vi "ADC Initialize Virtual Channels.vi"(8 "error in":errorcluster, 10 "Reset? (False)":bool, 11 "adc session in":T1={"niScope"={"channel cfg"=[], "sessions"=[], "multi cards"=FALSE, "channels"=0, "type"=enum."n/a", "memory [B/chn]"=0, "ext. clock [Hz]"=0.0, "samples count"=0, "use streaming"=FALSE, "proc setup"={"packet size [smpl]"=0, "current timeout [s]"=0.0, "blk2blk timeout [s]"=0.0, "event time"=timestamp(0 s since 1904-01-01), "temp sampl T [s]"=0.0, "data queue"=refnum, "stop notifier"=refnum, "proc ref"=refnum}, "sample width [B]"=0, "ranges [V]"=[], "trigger setup"={"coupling"=1, "level [V]"=0.0, "slope"=0, "mode"=enum."Immediate", "pre-trigger [%]"=0.0}, "fs [Hz]"=0.0, "bitres [bit]"=0, "clock source"=enum."VAL_NO_SOURCE"}, "3458A"={"channels"=[], "sync unit"={"VISA"="", "type"=enum."Picotest U6200A"}, "awg unit"={"type"=enum."Agilent 331xxA to 332xxA", "VISA"="", "enable 10MHz ref"=FALSE, "cmi ckd2"={"VISA"="", "clock source"=enum."Auto", "manual ref clk"=FALSE, "ref clock [Hz]"=0.0, "div mode"=enum."Set divisor directly"}, "cmi sync v3"={"VISA"="", "baud rate [bd/s]"=115200, "source"=enum."Auto", "hv range"=enum."1kV", "fsrc is fixed"=FALSE, "fsrc [Hz]"=10000000.0, "freq integ [s]"=1.0, "freq filter"=5, "trig level"=enum."TTL 5V", "chn1 mode"=enum."Source divider", "chn1 level"=enum."Positive 5V", "chn2 mode"=enum."Source divider", "chn2 level"=enum."Positive 5V", "chn2 div"=1, "chn3 mode"=enum."Chn 1 Active", "chn3 level"=enum."Positive 5V", "chn1 div entry"=enum."Calculate nearest divisor from measured fx", "chn1 dev limit [%]"=1.0, "chn1 check dev"=FALSE}, "trigger"={"source"=enum."Immediate", "slope"=enum."POS", "coupling"=enum."DC", "level [V]"=0.0, "hysteresis [V]"=0.0, "pre-trigger [%]"=0.0}, "HMF2500 cfg"={"Baud Rate"=9600, "Parity"=0, "Data Bits"=8, "Flow Control"=4}}, "sync mode"=enum."MASTER-SLAVE, MASTER clocked by TIMER", "streaming mode"=FALSE, "idn mode"=enum."Auto", "sampling mode"=enum."DCV", "sample memory [B]"=0, "proc setup"={"channel id"=0, "packet size [smpl]"=0, "current timeout [s]"=0.0, "blk2blk timeout [s]"=0.0, "event time"=timestamp(0 s since 1904-01-01), "stop notifier"=refnum, "data queues"=[], "proc refs"=[], "bus semaphore"=refnum}, "sample size [B]"=0, "sample count"=0, "aux data"={"channel id"=0, "valid?"=[], "gain [V]"=[], "timestamp [s]"=[], "Ts [s]"=0.0, "abs timestamp"=timestamp(0 s since 1904-01-01), "t [deg C]"=[], "multiplex timestamp [s]"=-1.0, "only multiplex?"=FALSE, "multiplex smpl offset"=0, "overflow?"=FALSE}, "ranges [V]"=[], "aperture [s]"=0.0, "LEVEL trigger"={"edge"=enum."POS", "level [V]"=0.0, "coupling"=enum."DC"}, "trigger mode"=enum."AUTO", "measure temp.?"=FALSE, "disp mesages"=[], "shared bus?"=FALSE, "disable display?"=FALSE, "aper mode"=enum."Manual", "aper rules"=[], "multiplex"={"cycles"=0, "delay [s]"=0.0, "enabled"=FALSE, "overhead [s]"=1.0, "tot smpls"=0, "sub-rec"=0, "overhead [%]"=0.0, "emulated"=FALSE}, "F8588 lpf"=enum."Off", "F8588 pll"=enum."Off", "F8588 couple"=enum."DC, auto", "fs"={"freq mode"=enum."fs or Ts", "fs [Hz]"=0.0, "fref [Hz]"=0.0, "mul"=0.0, "div"=0.0}, "fs mode"=enum."fs or Ts"}, "dsdll"={"dsdll"={"dsdll path"=path "", "dsdll handle"=[], "output devices"=[], "capture devices"=[]}, "channels"=0, "device id"=0, "channel idns"=[], "proc setup"={"packet size [smpl]"=0, "current timeout [s]"=0.0, "blk2blk timeout [s]"=0.0, "event time"=timestamp(0 s since 1904-01-01), "data queue"=refnum, "stop notifier"=refnum, "proc ref"=refnum}, "samples count"=0, "fs [Hz]"=0.0}, "type"=enum."niScope", "channel idn str"=[], "aux instr idn str"=[], "modified?"=FALSE, "simadc"={"channels"=[], "range [V]"=0.0, "Ts step [s]"=0.0, "time [s]"=0.0, "fs [Hz]"=0.0, "count"=0, "smpl offset"=0, "set count"=0, "bit res"=0}, "force rst?"=FALSE, "exit mode"=enum."Immediate reset", "exit dly"=0.0, "exit tmr"=timestamp(0 s since 1904-01-01), "busy?"=FALSE, "accessed?"=FALSE, "multiplex"={"Type"=enum."Dummy", "gen com ssn"={"visa"="", "primary"=enum."None", "secondary"=enum."None", "channels"=[]}, "delay before [s]"=0.0, "delay post [s]"=0.0, "sequence"=[], "enabled"=FALSE, "ref timestamp [s]"=0.0, "idn string"="", "dev niScope"="", "niScope idx"=0, "QPMX ssn"={"visa"="", "switch mode"=enum."Switched by TWM", "sequence"=[], "timing delays"=[], "polarity"=enum."Positive", "ss delay (s)"=2.0, "internal timer (s)"=1.0, "Last loaded sequence file"=path "", "startup delay (s)"=2.0}, "VISA mux ssn"={"VISA"="", "paths"=[], "idn command"="", "serial cfg"={"Baud rate"=9600, "Data bits"=8, "Parity"=0, "Stop bits"=10, "Flow control"=0, "End Mode Read"=enum."None", "End Mode Write"=enum."None", "Term character"=0, "Term enable"=FALSE}}}, "keysight dso"={"VISA"="", "channels"=[], "bw limit [Hz]"=0.0, "resolution"=enum."Basic", "trig noise reject"=enum."Normal", "N"=0, "trigger config"={"trigger source"=enum."Immediate", "trigger slope"=enum."Negative", "level [V]"=0.0, "hysteresis [V]"=0.001, "pre-trig [%]"=50}, "fs [Hz]"=0.0, "timeout stop"=timestamp(0 s since 1904-01-01), "waiting for opc"=FALSE, "fetch offset [smpl]"=0, "abs timestamp"=timestamp(0 s since 1904-01-01), "ranges [V]"=[], "decimation"=1.0, "ext ref"=FALSE, "emulate aperture"=FALSE, "model"=enum."DSO91304"}, "cdaq"={"mclk [Hz]"=12800000.0, "ADC task"="", "mclk reference"="", "fs [Hz]"=50000.0, "queue adc cmd"=refnum, "queue adc data"=refnum, "adc proc ref"=refnum, "channels"=[], "last channels"=[], "timeout"=timestamp(0 s since 1904-01-01), "N"=1000, "mclk mode"=enum."Free running", "ext mclk source"=""}, "ignore overload"=FALSE, "ADS127L21"={"VISA"="", "chn list"=[], "record size"=0, "phys. channels"=0, "adc fifo size"=0, "channels"=[], "ext refclk?"=FALSE, "fs [Hz]"=0.0, "ext refclk [Hz]"=0.0, "meas refclk [Hz]"=0.0, "EXTOUT mode"=enum."ADCCLK", "EXTOUT polarity"=enum."NORM", "EXTOUT divisor"=0}} {"ADS127L21"."channels"."Channel" min=1 max=8 step=1; "cdaq"."last channels"."Channel id" min=0 step=1; "cdaq"."channels"."Channel id" min=0 step=1; "keysight dso"."decimation" min=1.0; "keysight dso"."bw limit [Hz]" format="%#_6p"; "keysight dso"."channels"."Offset [V]" format="%#_6p"; "keysight dso"."channels"."Range [Vpk]" min=0.0 format="%#_6p"; "keysight dso"."channels"."Channel" min=1; "multiplex"."VISA mux ssn"."serial cfg"."Flow control" items=["None", "XON/XOFF", "CTS/RTS", "XON/XOFF + CTS/RTS", "DTR/DSR", "XON/XOFF + DTR/DSR"]; "multiplex"."VISA mux ssn"."serial cfg"."Stop bits" items=["1 bit"=10, "1.5 bits"=15, "2 bits"=20]; "multiplex"."VISA mux ssn"."serial cfg"."Parity" items=["None", "Odd", "Even", "Mark", "Space"]; "multiplex"."VISA mux ssn"."serial cfg"."Data bits" items=["5 bits"=5, "6 bits"=6, "7 bits"=7, "8 bits"=8]; "multiplex"."VISA mux ssn"."serial cfg"."Baud rate" items=["150 Bd"=150, "300 Bd"=300, "600 Bd"=600, "1200 Bd"=1200, "2400 Bd"=2400, "4800 Bd"=4800, "9600 Bd"=9600, "19.2 kBd"=19200, "38.4 kBd"=38400, "57.6 kBd"=57600, "115.2 kBd"=115200]; "multiplex"."QPMX ssn"."startup delay (s)" min=0.0 step=1.0; "multiplex"."QPMX ssn"."internal timer (s)" min=0.0 step=1.0; "multiplex"."QPMX ssn"."ss delay (s)" min=0.0 step=1.0; "multiplex"."QPMX ssn"."timing delays" min=1 max=255 step=1; "3458A"."awg unit"."HMF2500 cfg"."Flow Control" items=["None", "XON/XOFF", "RTS/CTS", "XON/XOFF & RTS/CTS", "DTR/DSR", "XON/XOFF & DTR/DSR"]; "3458A"."awg unit"."HMF2500 cfg"."Data Bits" items=["7"=7, "8"=8]; "3458A"."awg unit"."HMF2500 cfg"."Parity" items=["None", "Odd", "Even", "Mark", "Space"]; "3458A"."awg unit"."HMF2500 cfg"."Baud Rate" items=["300"=300, "600"=600, "1200"=1200, "2400"=2400, "4800"=4800, "9600"=9600, "19200"=19200]; "3458A"."awg unit"."cmi sync v3"."chn2 div" min=1 max=100000000 step=1; "3458A"."awg unit"."cmi sync v3"."fsrc [Hz]" format="%_8p"; "3458A"."channels"."Range [Vpk]" min=0.0; "niScope"."trigger setup"."pre-trigger [%]" format="%.2f"; "niScope"."trigger setup"."level [V]" format="%.2f"; "niScope"."trigger setup"."coupling" items=["AC"=0, "DC"=1, "HF Reject"=3, "LF Reject"=4, "AC Plus HF Reject"=1001]; "niScope"."channel cfg"."Range [Vpk]" min=0.0; "niScope"."channel cfg"."Channel" min=0}) -> (0 "error out":errorcluster, 1 "aux instr. idn strings":string[](array[string]), 2 "channel idn strings":string[](array[string]), 3 "adc session out":T1={"niScope"={"channel cfg"=[], "sessions"=[], "multi cards"=FALSE, "channels"=0, "type"=enum."n/a", "memory [B/chn]"=0, "ext. clock [Hz]"=0.0, "samples count"=0, "use streaming"=FALSE, "proc setup"={"packet size [smpl]"=0, "current timeout [s]"=0.0, "blk2blk timeout [s]"=0.0, "event time"=timestamp(0 s since 1904-01-01), "temp sampl T [s]"=0.0, "data queue"=refnum, "stop notifier"=refnum, "proc ref"=refnum}, "sample width [B]"=0, "ranges [V]"=[], "trigger setup"={"coupling"=1, "level [V]"=0.0, "slope"=0, "mode"=enum."Immediate", "pre-trigger [%]"=0.0}, "fs [Hz]"=0.0, "bitres [bit]"=0, "clock source"=enum."VAL_NO_SOURCE"}, "3458A"={"channels"=[], "sync unit"={"VISA"="", "type"=enum."Picotest U6200A"}, "awg unit"={"type"=enum."Agilent 331xxA to 332xxA", "VISA"="", "enable 10MHz ref"=FALSE, "cmi ckd2"={"VISA"="", "clock source"=enum."Auto", "manual ref clk"=FALSE, "ref clock [Hz]"=0.0, "div mode"=enum."Set divisor directly"}, "cmi sync v3"={"VISA"="", "baud rate [bd/s]"=115200, "source"=enum."Auto", "hv range"=enum."1kV", "fsrc is fixed"=FALSE, "fsrc [Hz]"=10000000.0, "freq integ [s]"=1.0, "freq filter"=5, "trig level"=enum."TTL 5V", "chn1 mode"=enum."Source divider", "chn1 level"=enum."Positive 5V", "chn2 mode"=enum."Source divider", "chn2 level"=enum."Positive 5V", "chn2 div"=1, "chn3 mode"=enum."Chn 1 Active", "chn3 level"=enum."Positive 5V", "chn1 div entry"=enum."Calculate nearest divisor from measured fx", "chn1 dev limit [%]"=1.0, "chn1 check dev"=FALSE}, "trigger"={"source"=enum."Immediate", "slope"=enum."POS", "coupling"=enum."DC", "level [V]"=0.0, "hysteresis [V]"=0.0, "pre-trigger [%]"=0.0}, "HMF2500 cfg"={"Baud Rate"=9600, "Parity"=0, "Data Bits"=8, "Flow Control"=4}}, "sync mode"=enum."MASTER-SLAVE, MASTER clocked by TIMER", "streaming mode"=FALSE, "idn mode"=enum."Auto", "sampling mode"=enum."DCV", "sample memory [B]"=0, "proc setup"={"channel id"=0, "packet size [smpl]"=0, "current timeout [s]"=0.0, "blk2blk timeout [s]"=0.0, "event time"=timestamp(0 s since 1904-01-01), "stop notifier"=refnum, "data queues"=[], "proc refs"=[], "bus semaphore"=refnum}, "sample size [B]"=0, "sample count"=0, "aux data"={"channel id"=0, "valid?"=[], "gain [V]"=[], "timestamp [s]"=[], "Ts [s]"=0.0, "abs timestamp"=timestamp(0 s since 1904-01-01), "t [deg C]"=[], "multiplex timestamp [s]"=-1.0, "only multiplex?"=FALSE, "multiplex smpl offset"=0, "overflow?"=FALSE}, "ranges [V]"=[], "aperture [s]"=0.0, "LEVEL trigger"={"edge"=enum."POS", "level [V]"=0.0, "coupling"=enum."DC"}, "trigger mode"=enum."AUTO", "measure temp.?"=FALSE, "disp mesages"=[], "shared bus?"=FALSE, "disable display?"=FALSE, "aper mode"=enum."Manual", "aper rules"=[], "multiplex"={"cycles"=0, "delay [s]"=0.0, "enabled"=FALSE, "overhead [s]"=1.0, "tot smpls"=0, "sub-rec"=0, "overhead [%]"=0.0, "emulated"=FALSE}, "F8588 lpf"=enum."Off", "F8588 pll"=enum."Off", "F8588 couple"=enum."DC, auto", "fs"={"freq mode"=enum."fs or Ts", "fs [Hz]"=0.0, "fref [Hz]"=0.0, "mul"=0.0, "div"=0.0}, "fs mode"=enum."fs or Ts"}, "dsdll"={"dsdll"={"dsdll path"=path "", "dsdll handle"=[], "output devices"=[], "capture devices"=[]}, "channels"=0, "device id"=0, "channel idns"=[], "proc setup"={"packet size [smpl]"=0, "current timeout [s]"=0.0, "blk2blk timeout [s]"=0.0, "event time"=timestamp(0 s since 1904-01-01), "data queue"=refnum, "stop notifier"=refnum, "proc ref"=refnum}, "samples count"=0, "fs [Hz]"=0.0}, "type"=enum."niScope", "channel idn str"=[], "aux instr idn str"=[], "modified?"=FALSE, "simadc"={"channels"=[], "range [V]"=0.0, "Ts step [s]"=0.0, "time [s]"=0.0, "fs [Hz]"=0.0, "count"=0, "smpl offset"=0, "set count"=0, "bit res"=0}, "force rst?"=FALSE, "exit mode"=enum."Immediate reset", "exit dly"=0.0, "exit tmr"=timestamp(0 s since 1904-01-01), "busy?"=FALSE, "accessed?"=FALSE, "multiplex"={"Type"=enum."Dummy", "gen com ssn"={"visa"="", "primary"=enum."None", "secondary"=enum."None", "channels"=[]}, "delay before [s]"=0.0, "delay post [s]"=0.0, "sequence"=[], "enabled"=FALSE, "ref timestamp [s]"=0.0, "idn string"="", "dev niScope"="", "niScope idx"=0, "QPMX ssn"={"visa"="", "switch mode"=enum."Switched by TWM", "sequence"=[], "timing delays"=[], "polarity"=enum."Positive", "ss delay (s)"=2.0, "internal timer (s)"=1.0, "Last loaded sequence file"=path "", "startup delay (s)"=2.0}, "VISA mux ssn"={"VISA"="", "paths"=[], "idn command"="", "serial cfg"={"Baud rate"=9600, "Data bits"=8, "Parity"=0, "Stop bits"=10, "Flow control"=0, "End Mode Read"=enum."None", "End Mode Write"=enum."None", "Term character"=0, "Term enable"=FALSE}}}, "keysight dso"={"VISA"="", "channels"=[], "bw limit [Hz]"=0.0, "resolution"=enum."Basic", "trig noise reject"=enum."Normal", "N"=0, "trigger config"={"trigger source"=enum."Immediate", "trigger slope"=enum."Negative", "level [V]"=0.0, "hysteresis [V]"=0.001, "pre-trig [%]"=50}, "fs [Hz]"=0.0, "timeout stop"=timestamp(0 s since 1904-01-01), "waiting for opc"=FALSE, "fetch offset [smpl]"=0, "abs timestamp"=timestamp(0 s since 1904-01-01), "ranges [V]"=[], "decimation"=1.0, "ext ref"=FALSE, "emulate aperture"=FALSE, "model"=enum."DSO91304"}, "cdaq"={"mclk [Hz]"=12800000.0, "ADC task"="", "mclk reference"="", "fs [Hz]"=50000.0, "queue adc cmd"=refnum, "queue adc data"=refnum, "adc proc ref"=refnum, "channels"=[], "last channels"=[], "timeout"=timestamp(0 s since 1904-01-01), "N"=1000, "mclk mode"=enum."Free running", "ext mclk source"=""}, "ignore overload"=FALSE, "ADS127L21"={"VISA"="", "chn list"=[], "record size"=0, "phys. channels"=0, "adc fifo size"=0, "channels"=[], "ext refclk?"=FALSE, "fs [Hz]"=0.0, "ext refclk [Hz]"=0.0, "meas refclk [Hz]"=0.0, "EXTOUT mode"=enum."ADCCLK", "EXTOUT polarity"=enum."NORM", "EXTOUT divisor"=0}} {"ADS127L21"."channels"."Channel" min=1 max=8 step=1; "cdaq"."last channels"."Channel id" min=0 step=1; "cdaq"."channels"."Channel id" min=0 step=1; "keysight dso"."decimation" min=1.0; "keysight dso"."bw limit [Hz]" format="%#_6p"; "keysight dso"."channels"."Offset [V]" format="%#_6p"; "keysight dso"."channels"."Range [Vpk]" min=0.0 format="%#_6p"; "keysight dso"."channels"."Channel" min=1; "multiplex"."VISA mux ssn"."serial cfg"."Flow control" items=["None", "XON/XOFF", "CTS/RTS", "XON/XOFF + CTS/RTS", "DTR/DSR", "XON/XOFF + DTR/DSR"]; "multiplex"."VISA mux ssn"."serial cfg"."Stop bits" items=["1 bit"=10, "1.5 bits"=15, "2 bits"=20]; "multiplex"."VISA mux ssn"."serial cfg"."Parity" items=["None", "Odd", "Even", "Mark", "Space"]; "multiplex"."VISA mux ssn"."serial cfg"."Data bits" items=["5 bits"=5, "6 bits"=6, "7 bits"=7, "8 bits"=8]; "multiplex"."VISA mux ssn"."serial cfg"."Baud rate" items=["150 Bd"=150, "300 Bd"=300, "600 Bd"=600, "1200 Bd"=1200, "2400 Bd"=2400, "4800 Bd"=4800, "9600 Bd"=9600, "19.2 kBd"=19200, "38.4 kBd"=38400, "57.6 kBd"=57600, "115.2 kBd"=115200]; "multiplex"."QPMX ssn"."startup delay (s)" min=0.0 step=1.0; "multiplex"."QPMX ssn"."internal timer (s)" min=0.0 step=1.0; "multiplex"."QPMX ssn"."ss delay (s)" min=0.0 step=1.0; "multiplex"."QPMX ssn"."timing delays" min=1 max=255 step=1; "3458A"."awg unit"."HMF2500 cfg"."Flow Control" items=["None", "XON/XOFF", "RTS/CTS", "XON/XOFF & RTS/CTS", "DTR/DSR", "XON/XOFF & DTR/DSR"]; "3458A"."awg unit"."HMF2500 cfg"."Data Bits" items=["7"=7, "8"=8]; "3458A"."awg unit"."HMF2500 cfg"."Parity" items=["None", "Odd", "Even", "Mark", "Space"]; "3458A"."awg unit"."HMF2500 cfg"."Baud Rate" items=["300"=300, "600"=600, "1200"=1200, "2400"=2400, "4800"=4800, "9600"=9600, "19200"=19200]; "3458A"."awg unit"."cmi sync v3"."chn2 div" min=1 max=100000000 step=1; "3458A"."awg unit"."cmi sync v3"."fsrc [Hz]" format="%_8p"; "3458A"."channels"."Range [Vpk]" min=0.0; "niScope"."trigger setup"."pre-trigger [%]" format="%.2f"; "niScope"."trigger setup"."level [V]" format="%.2f"; "niScope"."trigger setup"."coupling" items=["AC"=0, "DC"=1, "HF Reject"=3, "LF Reject"=4, "AC Plus HF Reject"=1001]; "niScope"."channel cfg"."Range [Vpk]" min=0.0; "niScope"."channel cfg"."Channel" min=0}, 4 "all instruments idn strings":string[](array[string]), 6 "multiplexer idn string":string)   [LabVIEW 2020]
doc: "Initialize ADC virtual channels. Initializes all intruments related to the virtual digitizer. It also reads identifications and some parameters needed for operation of the virtual ADC library. The VI modifies ADC session so don't throw away ADC session out!\n\nNote this VI also automatically opens a multiplexer if it is enabled. If so, it will create another additional virtual channels for each multiplexer sequence item."
uses:
  ADC Session.ctl
  drivers/niScope/niScope Session.ctl
  drivers/niScope/niScope Virtual Channel Config.ctl
  drivers/niScope/niScope Virtual Channel Mode.ctl
  drivers/niScope/niScope Virtual Channel Input Z.ctl
  drivers/niScope/niScope Virtual Channel Coupling.ctl
  drivers/niScope/niScope Type.ctl
  drivers/niScope/niScope Digitizing Process Options.ctl
  drivers/niScope/niScope Data Packet.ctl
  drivers/niScope/niScope Trigger Setup.ctl
  <instrlib>/niScope/Controls/niScope trigger coupling.ctl
  <instrlib>/niScope/Controls/niScope trigger slope.ctl
  drivers/niScope/niScope Reference Clock.ctl
  drivers/DMM/3458A Digitizer Session.ctl
  drivers/DMM/3458A Virtual Channel Config.ctl
  drivers/Counter/Counter Session.ctl
  drivers/Counter/Counter Type.ctl
  drivers/AWG/AWG Session.ctl
  drivers/AWG/AWG Type.ctl
  drivers/AWG/CMI Clock Divider v2/CMI ckd2 Session.ctl
  drivers/AWG/CMI Clock Divider v2/CMI ckd2 Source Mode.ctl
  drivers/AWG/CMI Clock Divider v2/CMI ckd2 Divisor Mode.ctl
  drivers/AWG/CMI Sync V3/CMI Sync V3 session.ctl
  drivers/AWG/CMI Sync V3/Configure/CMI Sync V3 Reference Clock Source.ctl
  drivers/AWG/CMI Sync V3/Configure/CMI Sync V3 HV input Range.ctl
  drivers/AWG/CMI Sync V3/Configure/CMI Sync V3 Trigger Input Level.ctl
  drivers/AWG/CMI Sync V3/Configure/CMI Sync V3 Channel 1 Mode.ctl
  drivers/AWG/CMI Sync V3/Configure/CMI Sync V3 Channel Output Levels.ctl
  drivers/AWG/CMI Sync V3/Configure/CMI Sync V3 Channel 2 Mode.ctl
  drivers/AWG/CMI Sync V3/Configure/CMI Sync V3 Channel 3 Mode.ctl
  drivers/AWG/CMI Sync V3/Configure/CMI Sync V3 Channel 1 Divisor Entry Mode.ctl
  ADC Trig Config.ctl
  ADC Trig Mode Source.ctl
  ADC Trig Slope.ctl
  ADC Trig Coupling.ctl
  drivers/AWG/RaS HMF2500/HMF2500 Config.ctl
  drivers/DMM/3458A Sync Mode.ctl
  drivers/DMM/3458A Idn Mode.ctl
  drivers/DMM/3458A Digitizing Low Levels/Configure/Sampling Mode.ctl
  drivers/DMM/3458A Digitizing Process Options.ctl
  drivers/DMM/3458A Data Packet.ctl
  drivers/DMM/3458A Aux Record Data.ctl
  drivers/DMM/3458A Digitizing Low Levels/Configure/Level Setup.ctl
  drivers/DMM/3458A Digitizing Low Levels/Configure/First Sample Trigger.ctl
  drivers/DMM/3458A Aperture Selection Mode.ctl
  drivers/DMM/3458A Multiplexing Config.ctl
  drivers/Fluke 8588A/F8588A Low Pass Filter.ctl
  drivers/Fluke 8588A/F8588A Phase Lock.ctl
  drivers/Fluke 8588A/F8588A Coupling.ctl
  drivers/DMM/3458A Sampling Rate.ctl
  drivers/AWG/AWG Clock Setup Mode.ctl
  drivers/DMM/3458A Sample Rate Mode.ctl
  drivers/dsdll/DSDLL Session.ctl
  drivers/dsdll/dsdll/dsdll_instance.ctl
  drivers/dsdll/dsdll/dsdll_device_record.ctl
  drivers/dsdll/DSDLL Process Config.ctl
  drivers/dsdll/DSDLL Data Packet.ctl
  ADC Type.ctl
  drivers/simulated_adc/SimAdc Config.ctl
  drivers/simulated_adc/SimAdc Channel Cfg.ctl
  ADC On Close Action.ctl
  Multiplexer/MPX Session.ctl
  Multiplexer/MPX Type.ctl
  drivers/Multiplexers/Generic COM/GCOMM Session.ctl
  drivers/Multiplexers/Generic COM/GCOMM Signal.ctl
  drivers/Multiplexers/Generic COM/GCOMM Virtual Channel.ctl
  drivers/Multiplexers/Generic COM/GCOMM Logic State.ctl
  drivers/Multiplexers/Generic COM/QPMX Session.ctl
  drivers/Multiplexers/QPMX/QPMX switch mode.ctl
  drivers/Multiplexers/QPMX/QPMX polarity.ctl
  drivers/Multiplexers/Generic VISA commands/GVISA Mux Session.ctl
  drivers/Multiplexers/Generic VISA commands/GVISA Mux Path Entry.ctl
  drivers/Multiplexers/Generic VISA commands/met_serial_setup.ctl
  drivers/Agilent DSO 90000/Virtual Digitizer/KeDSO session.ctl
  drivers/Agilent DSO 90000/Virtual Digitizer/KeDSO Virtual Channel.ctl
  drivers/Agilent DSO 90000/Virtual Digitizer/KeDSO High Resolution Mode.ctl
  drivers/Agilent DSO 90000/Virtual Digitizer/KeDSO Trigger Setup.ctl
  drivers/Agilent DSO 90000/Virtual Digitizer/KeDSO Trigger Source.ctl
  drivers/Agilent DSO 90000/Public/Utility/DSO type.ctl
  drivers/cdaq/cDAQ Session.ctl
  drivers/cdaq/low_level_old/cdaq_anal_adc_command.ctl
  drivers/cdaq/low_level_old/cdaq_anal_adc_data.ctl
  drivers/cdaq/cDAQ Virtual Channel.ctl
  drivers/cdaq/cDAQ Master Clock Mode.ctl
  drivers/CMI_ADS127L21/CMI ADS127L21 - Session.ctl
  drivers/CMI_ADS127L21/CMI ADS127L21 - Record Channel.ctl
  drivers/CMI_ADS127L21/CMI ADS127L21 - Input Range.ctl
  drivers/CMI_ADS127L21/CMI ADS127L21 - Input Mode.ctl
  drivers/CMI_ADS127L21/CMI ADS127L21 - Input Impedance.ctl
  drivers/CMI_ADS127L21/CMI ADS127L21 - EXTOUT Mode.ctl
  drivers/CMI_ADS127L21/CMI ADS127L21 - EXTOUT Polarity.ctl
  drivers/DMM/3458A Virtual Digitizer.lvlib
  drivers/niScope/niScope Virtual Digitizer.lvlib
  drivers/dsdll/DSDLL Virtual Digitizer.lvlib
  <vilib>/ErrorRing/Error Ring.xnode
  <vilib>/Utility/error.llb/Error Cluster From Error Code.vi
  drivers/Counter/Counter.lvlib
  drivers/AWG/AWG.lvlib
  drivers/DMM/3458A Digitizing Low Levels/3458A Digitizing Low Levels.lvlib
  drivers/dsdll/dsdll/dsdll.lvlib
  drivers/AWG/CMI Sync V3/CMI Sync Unit V3.lvlib
  drivers/Agilent DSO 90000/Agilent 90000 Series.lvlib
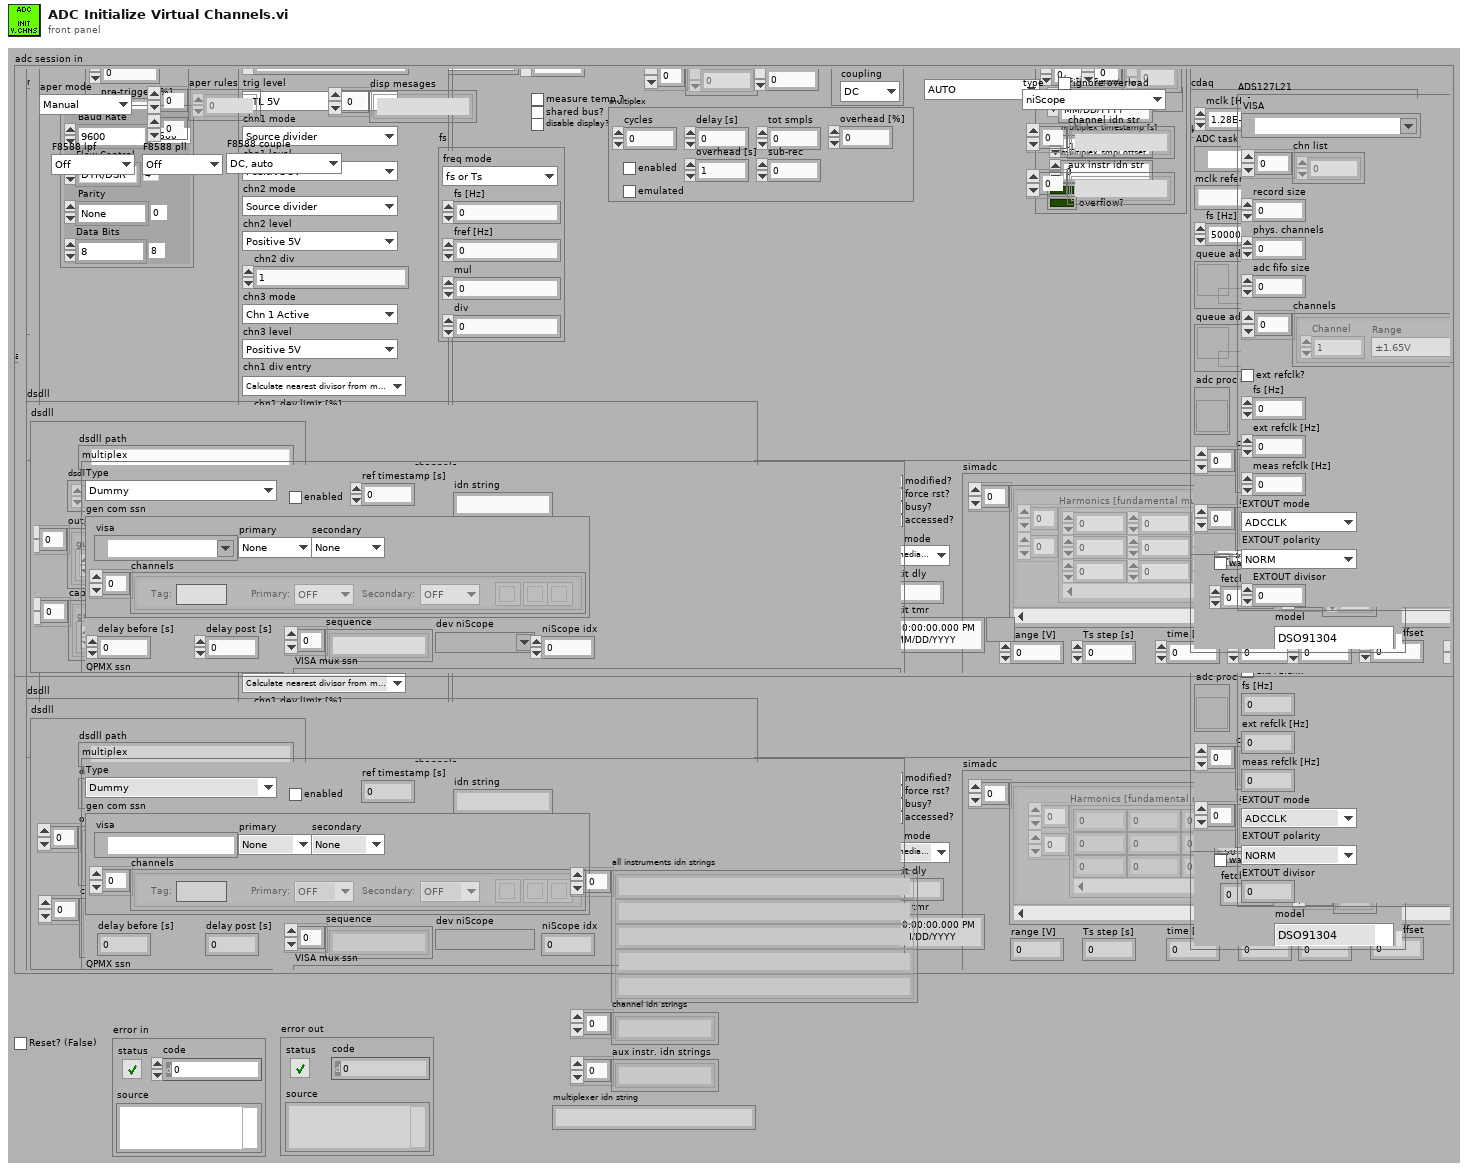
[diagram p1: front panel]
types:
  T1 = typedef "ADC Session.ctl" = cluster{"niScope":T2, "3458A":T13, "dsdll":T52, "type":T56, "channel idn str":string[], "aux instr idn str":string[], "modified?":bool, "simadc":T57, "force rst?":bool, "exit mode":T59, "exit dly":dbl, "exit tmr":timestamp, "busy?":bool, "accessed?":bool, "multiplex":T60, "keysight dso":T72, "cdaq":T78, "ignore overload":bool, "ADS127L21":T81}
  T2 = typedef "niScope Virtual Digitizer.lvlib/niScope Session.ctl" = cluster{"channel cfg":T3[], "sessions":refnum<k20>[], "multi cards":bool, "channels":i32, "type":T7, "memory [B/chn]":i32, "ext. clock [Hz]":dbl, "samples count":i64, "use streaming":bool, "proc setup":T8, "sample width [B]":i32, "ranges [V]":dbl[], "trigger setup":T9, "fs [Hz]":dbl, "bitres [bit]":i32, "clock source":T12}
  T3 = typedef "niScope Virtual Digitizer.lvlib/niScope Virtual Channel Config.ctl" = cluster{"Address":refnum<k15>, "Channel":i32, "Mode":T4, "Input Z":T5, "Coupling":T6, "Range [Vpk]":dbl, "btn clr":bool, "btn up":bool, "btn down":bool}
  T4 = typedef "niScope Virtual Digitizer.lvlib/niScope Virtual Channel Mode.ctl" = enum16{"Single ended", "Unbal. differential", "Differential"}
  T5 = typedef "niScope Virtual Digitizer.lvlib/niScope Virtual Channel Input Z.ctl" = enum16{"1 MOhm", "50 Ohm"}
  T6 = typedef "niScope Virtual Digitizer.lvlib/niScope Virtual Channel Coupling.ctl" = enum16{"AC", "DC", "GND"}
  T7 = typedef "niScope Virtual Digitizer.lvlib/niScope Type.ctl" = enum16{"n/a", "5922"}
  T8 = typedef "niScope Virtual Digitizer.lvlib/niScope Digitizing Process Options.ctl" = cluster{"packet size [smpl]":i64, "current timeout [s]":dbl, "blk2blk timeout [s]":dbl, "event time":timestamp, "temp sampl T [s]":dbl, "data queue":refnum<queue>, "stop notifier":refnum<notifier>, "proc ref":refnum<vi>}
  T9 = typedef "niScope Virtual Digitizer.lvlib/niScope Trigger Setup.ctl" = cluster{"coupling":T10, "level [V]":dbl, "slope":T11, "mode":enum16{"Immediate", "External", "Level"}, "pre-trigger [%]":dbl}
  T10 = typedef "niScope trigger coupling.ctl" = u16
  T11 = typedef "niScope trigger slope.ctl" = i32
  T12 = typedef "niScope Virtual Digitizer.lvlib/niScope Reference Clock.ctl" = enum16{"VAL_NO_SOURCE", "VAL_CLK_IN", "VAL_PXI_CLOCK", "VAL_EXTERNAL"}
  T13 = typedef "3458A Virtual Digitizer.lvlib/3458A Digitizer Session.ctl" = cluster{"channels":T14[], "sync unit":T15, "awg unit":T17, "sync mode":T36, "streaming mode":bool, "idn mode":T37, "sampling mode":T38, "sample memory [B]":i32, "proc setup":T39, "sample size [B]":i32, "sample count":i32, "aux data":T41, "ranges [V]":dbl[], "aperture [s]":dbl, "LEVEL trigger":T42, "trigger mode":T43, "measure temp.?":bool, "disp mesages":string[], "shared bus?":bool, "disable display?":bool, "aper mode":T44, "aper rules":dbl[][], "multiplex":T45, "F8588 lpf":T46, "F8588 pll":T47, "F8588 couple":T48, "fs":T49, "fs mode":T51}
  T14 = typedef "3458A Virtual Digitizer.lvlib/3458A Virtual Channel Config.ctl" = cluster{"VISA":refnum<visa-resource-name>, "Range [Vpk]":dbl, "btn clr":bool, "btn up":bool, "btn down":bool, "F8588":bool, "F8588 guard":bool}
  T15 = typedef "Counter.lvlib/Counter Session.ctl" = cluster{"VISA":refnum<visa-resource-name>, "type":T16}
  T16 = typedef "Counter.lvlib/Counter Type.ctl" = enum16{"Picotest U6200A", "dummy"}
  T17 = typedef "AWG.lvlib/AWG Session.ctl" = cluster{"type":T18, "VISA":refnum<visa-resource-name>, "enable 10MHz ref":bool, "cmi ckd2":T19, "cmi sync v3":T22, "trigger":T31, "HMF2500 cfg":T35}
  T18 = typedef "AWG.lvlib/AWG Type.ctl" = enum16{"Agilent 331xxA to 332xxA", "Agilent 335xxA to 336xxA", "Tektronix AFG3101C", "R&S HMF25xx", "CMI Clock Divider v2", "CMI Sync Unit V3", "dummy"}
  T19 = typedef "AWG.lvlib/CMI ckd2 Session.ctl" = cluster{"VISA":refnum<visa-resource-name>, "clock source":T20, "manual ref clk":bool, "ref clock [Hz]":dbl, "div mode":T21}
  T20 = typedef "AWG.lvlib/CMI ckd2 Source Mode.ctl" = enum16{"Auto", "LF clock", "HF clock", "Internal"}
  T21 = typedef "AWG.lvlib/CMI ckd2 Divisor Mode.ctl" = enum16{"Set divisor directly", "Set divisor by frequency"}
  T22 = typedef "AWG.lvlib/CMI Sync Unit V3.lvlib/CMI Sync V3 session.ctl" = cluster{"VISA":refnum<visa-resource-name>, "baud rate [bd/s]":i32, "source":T23, "hv range":T24, "fsrc is fixed":bool, "fsrc [Hz]":dbl, "freq integ [s]":dbl, "freq filter":i32, "trig level":T25, "chn1 mode":T26, "chn1 level":T27, "chn2 mode":T28, "chn2 level":T27, "chn2 div":i32, "chn3 mode":T29, "chn3 level":T27, "chn1 div entry":T30, "chn1 dev limit [%]":dbl, "chn1 check dev":bool}
  T23 = typedef "AWG.lvlib/CMI Sync Unit V3.lvlib/CMI Sync V3 Reference Clock Source.ctl" = enum16{"Auto", "Internal", "Logic", "Sine", "HV"}
  T24 = typedef "AWG.lvlib/CMI Sync Unit V3.lvlib/CMI Sync V3 HV input Range.ctl" = enum16{"10V", "60V", "250V", "1kV"}
  T25 = typedef "AWG.lvlib/CMI Sync Unit V3.lvlib/CMI Sync V3 Trigger Input Level.ctl" = enum16{"LVCMOS 3V3", "TTL 5V"}
  T26 = typedef "AWG.lvlib/CMI Sync Unit V3.lvlib/CMI Sync V3 Channel 1 Mode.ctl" = enum16{"Source divider", "DDS absolute", "DDS ratio", "DDS ratio M/N"}
  T27 = typedef "AWG.lvlib/CMI Sync Unit V3.lvlib/CMI Sync V3 Channel Output Levels.ctl" = enum16{"Positive 3V3", "Negative 3V3", "Positive 5V", "Negative 5V"}
  T28 = typedef "AWG.lvlib/CMI Sync Unit V3.lvlib/CMI Sync V3 Channel 2 Mode.ctl" = enum16{"Source divider", "Chn 1 divide"}
  T29 = typedef "AWG.lvlib/CMI Sync Unit V3.lvlib/CMI Sync V3 Channel 3 Mode.ctl" = enum16{"Chn 1 Active", "Chn 2 Active", "Chn 1 Trigger", "Chn 2 Trigger", "Gate", "PPS", "10MHz"}
  T30 = typedef "AWG.lvlib/CMI Sync Unit V3.lvlib/CMI Sync V3 Channel 1 Divisor Entry Mode.ctl" = enum16{"Set divisor directly", "Calculate nearest divisor from measured fx"}
  T31 = typedef "ADC Trig Config.ctl" = cluster{"source":T32, "slope":T33, "coupling":T34, "level [V]":dbl, "hysteresis [V]":dbl, "pre-trigger [%]":dbl}
  T32 = typedef "ADC Trig Mode Source.ctl" = enum16{"Immediate", "External", "Level"}
  T33 = typedef "ADC Trig Slope.ctl" = enum16{"POS", "NEG"}
  T34 = typedef "ADC Trig Coupling.ctl" = enum16{"DC", "AC"}
  T35 = typedef "AWG.lvlib/HMF2500 Config.ctl" = cluster{"Baud Rate":u32, "Parity":u16, "Data Bits":u16, "Flow Control":u16}
  T36 = typedef "3458A Virtual Digitizer.lvlib/3458A Sync Mode.ctl" = enum16{"MASTER-SLAVE, MASTER clocked by TIMER", "MASTER-SLAVE, MASTER clocked by AWG", "ALL clocked by AWG", "MASTER-SLAVE, ALL clocked by TIMER", "ALL clocked by AWG with DFLL"}
  T37 = typedef "3458A Virtual Digitizer.lvlib/3458A Idn Mode.ctl" = enum16{"Auto", "Sequential (chn A, chn B, ...)", "From calibration string"}
  T38 = typedef "3458A Virtual Digitizer.lvlib/3458A Digitizing Low Levels.lvlib/Sampling Mode.ctl" = enum16{"DCV", "DSDC", "DSAC"}
  T39 = typedef "3458A Virtual Digitizer.lvlib/3458A Digitizing Process Options.ctl" = cluster{"channel id":i32, "packet size [smpl]":i32, "current timeout [s]":dbl, "blk2blk timeout [s]":dbl, "event time":timestamp, "stop notifier":refnum<notifier>, "data queues":refnum<queue>[], "proc refs":refnum<vi>[], "bus semaphore":T40}
  T40 = typedef "Semaphore RefNum" = refnum<k1>
  T41 = typedef "3458A Virtual Digitizer.lvlib/3458A Aux Record Data.ctl" = cluster{"channel id":i32, "valid?":bool[], "gain [V]":dbl[], "timestamp [s]":dbl[], "Ts [s]":dbl, "abs timestamp":timestamp, "t [deg C]":dbl[], "multiplex timestamp [s]":dbl, "only multiplex?":bool, "multiplex smpl offset":i64, "overflow?":bool}
  T42 = typedef "3458A Virtual Digitizer.lvlib/3458A Digitizing Low Levels.lvlib/Level Setup.ctl" = cluster{"edge":enum16{"POS", "NEG"}, "level [V]":dbl, "coupling":enum16{"DC", "AC"}}
  T43 = typedef "3458A Virtual Digitizer.lvlib/3458A Digitizing Low Levels.lvlib/First Sample Trigger.ctl" = enum16{"AUTO", "EXT", "SYN", "SGL", "HOLD", "LEVEL"}
  T44 = typedef "3458A Virtual Digitizer.lvlib/3458A Aperture Selection Mode.ctl" = enum16{"Manual", "Maximum", "Table"}
  T45 = typedef "3458A Virtual Digitizer.lvlib/3458A Multiplexing Config.ctl" = cluster{"cycles":i32, "delay [s]":dbl, "enabled":bool, "overhead [s]":dbl, "tot smpls":i64, "sub-rec":i32, "overhead [%]":dbl, "emulated":bool}
  T46 = typedef "F8588A Low Pass Filter.ctl" = enum16{"Off", "100 kHz", "3 MHz"}
  T47 = typedef "F8588A Phase Lock.ctl" = enum16{"Off", "1 MHz", "10 MHz"}
  T48 = typedef "F8588A Coupling.ctl" = enum16{"AC, 1 MOhm", "AC, 10 MOhm", "DC, 1 MOhm", "DC, 10 MOhm", "DC, auto"}
  T49 = typedef "3458A Virtual Digitizer.lvlib/3458A Sampling Rate.ctl" = cluster{"freq mode":T50, "fs [Hz]":dbl, "fref [Hz]":dbl, "mul":dbl, "div":dbl}
  T50 = typedef "AWG.lvlib/AWG Clock Setup Mode.ctl" = enum16{"fs or Ts", "fs or Ts with fref", "fref/N", "fref*M/N", "fref*Ratio"}
  T51 = typedef "3458A Sample Rate Mode.ctl" = enum16{"fs or Ts", "fs*M/N"}
  T52 = typedef "DSDLL Virtual Digitizer.lvlib/DSDLL Session.ctl" = cluster{"dsdll":T53, "channels":i32, "device id":i32, "channel idns":string[], "proc setup":T55, "samples count":i32, "fs [Hz]":dbl}
  T53 = typedef "dsdll.lvlib/dsdll_instance.ctl" = cluster{"dsdll path":path, "dsdll handle":u8[], "output devices":T54[], "capture devices":T54[]}
  T54 = typedef "dsdll.lvlib/dsdll_device_record.ctl" = cluster{"guid":u8[], "name":string}
  T55 = typedef "DSDLL Virtual Digitizer.lvlib/DSDLL Process Config.ctl" = cluster{"packet size [smpl]":i32, "current timeout [s]":dbl, "blk2blk timeout [s]":dbl, "event time":timestamp, "data queue":refnum<queue>, "stop notifier":refnum<notifier>, "proc ref":refnum<vi>}
  T56 = typedef "ADC Type.ctl" = enum16{"niScope", "3458A", "DirectSound DLL", "Keysight DSO", "cDAQ ADC", "CMI ADS127L21", "dummy"}
  T57 = typedef "SimAdc Config.ctl" = cluster{"channels":T58[], "range [V]":dbl, "Ts step [s]":dbl, "time [s]":dbl, "fs [Hz]":dbl, "count":i64, "smpl offset":i64, "set count":i64, "bit res":i32}
  T58 = typedef "SimAdc Channel Cfg.ctl" = cluster{"harmonics":dbl[][], "btn clear":bool, "noise":dbl, "fundamental [Hz]":dbl}
  T59 = typedef "ADC On Close Action.ctl" = enum16{"Immediate reset", "Delayed reset"}
  T60 = typedef "MPX Session.ctl" = cluster{"Type":T61, "gen com ssn":T62, "delay before [s]":dbl, "delay post [s]":dbl, "sequence":string[], "enabled":bool, "ref timestamp [s]":dbl, "idn string":string, "dev niScope":refnum<k15>, "niScope idx":i32, "QPMX ssn":T66, "VISA mux ssn":T69}
  T61 = typedef "MPX Type.ctl" = enum16{"Dummy", "Generic - COM port", "Generic - niScope PFI", "Generic - VISA commands", "QPMX"}
  T62 = typedef "GCOMM Session.ctl" = cluster{"visa":refnum<visa-resource-name>, "primary":T63, "secondary":T63, "channels":T64[]}
  T63 = typedef "GCOMM Signal.ctl" = enum16{"None", "DTR", "RTS"}
  T64 = typedef "GCOMM Virtual Channel.ctl" = cluster{"Primary:":T65, "Secondary:":T65, "btn clr":bool, "btn up":bool, "btn down":bool, "Tag:":string}
  T65 = typedef "GCOMM Logic State.ctl" = enum16{"OFF", "ON"}
  T66 = typedef "QPMX Session.ctl" = cluster{"visa":refnum<visa-resource-name>, "switch mode":T67, "sequence":bool[][], "timing delays":u32[], "polarity":T68, "ss delay (s)":dbl, "internal timer (s)":dbl, "Last loaded sequence file":path, "startup delay (s)":dbl}
  T67 = typedef "QPMX switch mode.ctl" = enum16{"Switched by TWM", "Switched by external clock", "Switched by internal clock"}
  T68 = typedef "QPMX polarity.ctl" = enum16{"Positive", "Negative"}
  T69 = typedef "GVISA Mux Session.ctl" = cluster{"VISA":refnum<visa-resource-name>, "paths":T70[], "idn command":string, "serial cfg":T71}
  T70 = typedef "GVISA Mux Path Entry.ctl" = cluster{"Tag:":string, "Command:":string, "btn clr":bool, "btn up":bool, "btn down":bool}
  T71 = typedef "met_serial_setup.ctl" = cluster{"Baud rate":i32, "Data bits":i32, "Parity":i32, "Stop bits":i32, "Flow control":i32, "End Mode Read":enum16{"None", "Last Bit", "TermChar"}, "End Mode Write":enum16{"None", "Last Bit", "TermChar"}, "Term character":u8, "Term enable":bool}
  T72 = typedef "KeDSO session.ctl" = cluster{"VISA":refnum<visa-resource-name>, "channels":T73[], "bw limit [Hz]":dbl, "resolution":T74, "trig noise reject":enum16{"Normal", "High Sensitivity"}, "N":i64, "trigger config":T75, "fs [Hz]":dbl, "timeout stop":timestamp, "waiting for opc":bool, "fetch offset [smpl]":i64, "abs timestamp":timestamp, "ranges [V]":dbl[], "decimation":dbl, "ext ref":bool, "emulate aperture":bool, "model":T77}
  T73 = typedef "KeDSO Virtual Channel.ctl" = cluster{"Channel":i32, "Range [Vpk]":dbl, "btn clr":bool, "btn up":bool, "btn down":bool, "Offset [V]":dbl, "Coupling":enum16{"DC", "DC50", "AC", "LFR1"}, "bw limit enab":bool}
  T74 = typedef "KeDSO High Resolution Mode.ctl" = enum16{"Basic", "High-res AUTO", "Min. 9-bits", "Min. 10-bits", "Min. 11-bits", "Min. 12-bits", "Fixed 11-bits", "Fixed 12-bits", "Fixed 13-bits", "Fixed 14-bits", "Fixed 15-bits", "Fixed 16-bits"}
  T75 = typedef "KeDSO Trigger Setup.ctl" = cluster{"trigger source":T76, "trigger slope":enum16{"Negative", "Positive", "Either"}, "level [V]":dbl, "hysteresis [V]":dbl, "pre-trig [%]":i32}
  T76 = typedef "KeDSO Trigger Source.ctl" = enum16{"Immediate", "Level", "AUX"}
  T77 = typedef "Agilent 90000 Series.lvlib/DSO type.ctl" = enum16{"DSO91304", "DSO91204", "DSO90804", "DSO90604", "DSO90404", "DSO90254", "DSA91304", "DSA91204", "DSA90804", "DSA90604", "DSA90404", "DSA90254", "DSO9104", "DSO9254", "DSO9404", "MSO9104", "MSO9254", "MSO9404", "MSO9064", "DSO9064", "DSOX91604", "DSOX92004", "DSOX92504", "DSOX92804", "DSOX93204", "DSO93004", "DSO9024H", "DSO9054H", "DSO9104H", "DSO9204H", "DSOS054A", "DSOS104A", "DSOS204A", "DSOS254A", "DSOS404A", "DSOS604A", "DSOS804A", "MSOS054A", "MSOS104A", "MSOS204A", "MSOS254A", "MSOS404A", "MSOS604A", "MSOS804A", "DSAX96204Q", "DSOX96204Q", "DSAX95004Q", "DSOX95004Q", "DSAX93304Q", "DSOX93304Q", "DSAX92504Q", "DSOX92504Q", "DSAX92004Q", "DSOX92004Q"}
  T78 = typedef "cDAQ Session.ctl" = cluster{"mclk [Hz]":dbl, "ADC task":refnum<k21>, "mclk reference":string, "fs [Hz]":dbl, "queue adc cmd":refnum<queue>, "queue adc data":refnum<queue>, "adc proc ref":refnum<vi>, "channels":T79[], "last channels":T79[], "timeout":timestamp, "N":i32, "mclk mode":T80, "ext mclk source":tag}
  T79 = typedef "cDAQ Virtual Channel.ctl" = cluster{"Device":tag, "Channel id":i32, "btn clr":bool, "btn up":bool, "btn down":bool}
  T80 = typedef "cDAQ Master Clock Mode.ctl" = enum16{"Free running", "Export master clock", "Import master clock"}
  T81 = typedef "CMI ADS127L21 - Session.ctl" = cluster{"VISA":refnum<visa-resource-name>, "chn list":i32[], "record size":i32, "phys. channels":i32, "adc fifo size":i32, "channels":T82[], "ext refclk?":bool, "fs [Hz]":dbl, "ext refclk [Hz]":dbl, "meas refclk [Hz]":dbl, "EXTOUT mode":T86, "EXTOUT polarity":T87, "EXTOUT divisor":i32}
  T82 = typedef "CMI ADS127L21 - Record Channel.ctl" = cluster{"Range":T83, "Channel":i32, "Mode":T84, "Impedance":T85}
  T83 = typedef "CMI ADS127L21 - Input Range.ctl" = enum16{"±1.65V", "±2V"}
  T84 = typedef "CMI ADS127L21 - Input Mode.ctl" = enum16{"Normal", "Inverted", "GND"}
  T85 = typedef "CMI ADS127L21 - Input Impedance.ctl" = enum16{"1M", "1k5"}
  T86 = typedef "CMI ADS127L21 - EXTOUT Mode.ctl" = enum16{"ADCCLK", "REFCLK", "SMPLCLK", "FIRST"}
  T87 = typedef "CMI ADS127L21 - EXTOUT Polarity.ctl" = enum16{"NORM", "INV"}
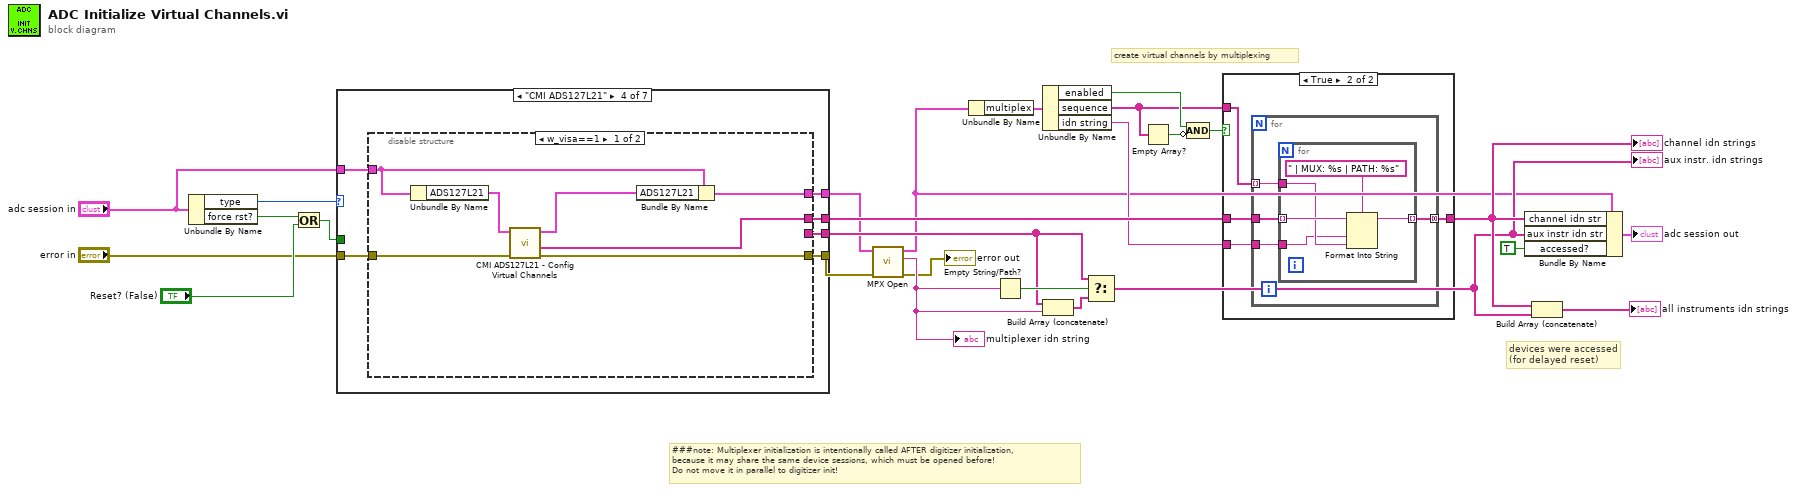
[diagram p0: block diagram]
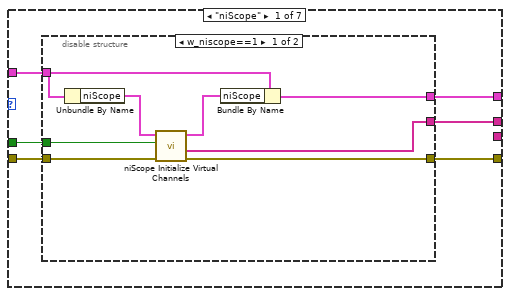
[diagram p3: hidden frame]
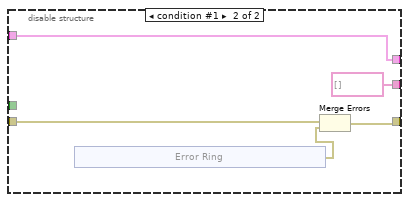
[diagram p4: hidden frame]
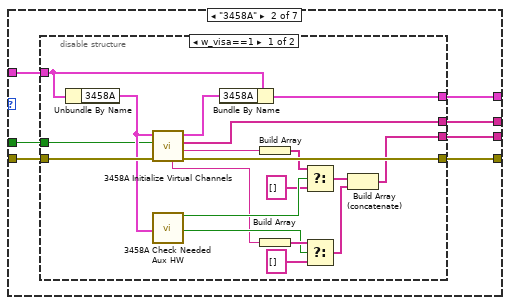
[diagram p5: hidden frame]
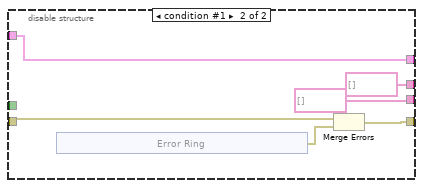
[diagram p6: hidden frame]
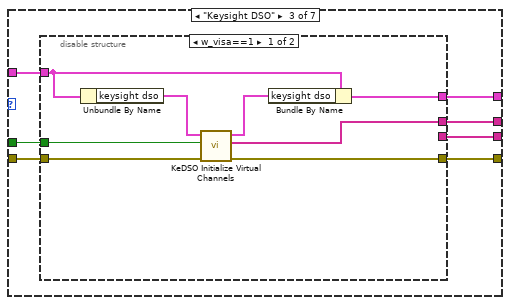
[diagram p7: hidden frame]
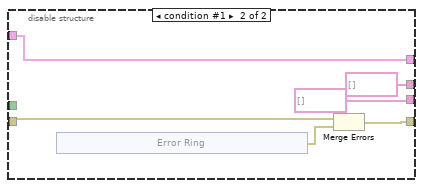
[diagram p8: hidden frame]
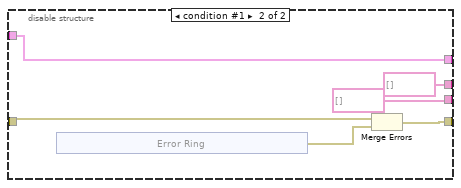
[diagram p9: hidden frame]
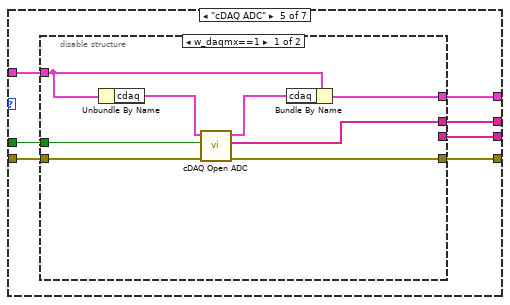
[diagram p10: hidden frame]
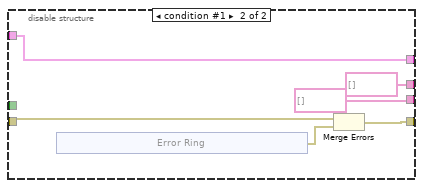
[diagram p11: hidden frame]
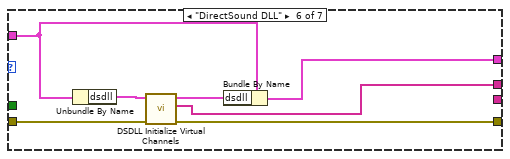
[diagram p12: hidden frame]
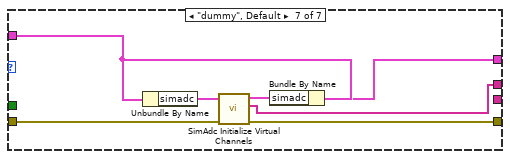
[diagram p13: hidden frame]
diagram:
  # "###note: Multiplexer initialization is intentionally called AFTER digitizer initialization,\nbecause it may share the same device sessions, which must be opened before!\nDo not move it in parallel to digitizer init!"
  # "create virtual channels by multiplexing"
  # "devices were accessed\n(for delayed reset)"
  n1 = Unbundle By Name("adc session in") -> ("type"=w26:T56, "force rst?"=w24:bool)
  n2 = Or(x=w24, y="Reset? (False)") -> (x .or. y?=w22:bool)
  n3 = case shown="\"CMI ADS127L21\"" w26 {
    tunnel: "error in" -> [w32 w57 w94 w119 w144 w170 w177]
    tunnel: "adc session in" -> [w31 w56 w93 w118 w143 w168 w174]
    tunnel: [w30 w55 w92 w117 w142 w165 w171] -> w2
    tunnel: [w29 w54 w91 w116 w141 w166 w176] -> w3
    tunnel: [w27 w53 w90 w115 w140 w164 w172] -> w13
    tunnel: [_ w52 w89 w114 w139 _ _] -> w9
    tunnel: w22 -> [w28 w51 w88 _ w138 _ _]
    frame "niScope" {
      n4 = disable-structure shown="w_niscope==1" {
        disable-tunnel: w32 -> [w40 w45]
        disable-tunnel: w31 -> [w38 w42]
        disable-tunnel: [w36 w42] -> w30
        disable-tunnel: [w35 w44] -> w29
        disable-tunnel: w28 -> [w34 _]
        disable-tunnel: [w33 string[] [] ("idn strings")] -> w27
        frame condition #0 (active) {
          n5 = Unbundle By Name(w38) -> ("niScope"=w39:T2)
          n6 = call "niScope Initialize Virtual Channels.vi"("error in"=w40, "Reset card (False)"=w34, "niScope in"=w39) -> ("error out"=w35:errorcluster, "idn strings"=w33:string[], "niScope out"=w37:T2)  [unwired: 5 in, 1 out]
          n7 = Bundle By Name(cluster=w38, "niScope"=w37) -> (w36:T1)
        }
        frame condition #1 {
          n8 = xnode "Error Ring"() -> ("error out"=w43:errorcluster)
          n9 = Merge Errors(w45, w43) -> (w44:errorcluster)
        }
      }
    }
    frame "3458A" {
      n10 = disable-structure shown="w_visa==1" {
        disable-tunnel: w57 -> [w76 w82]
        disable-tunnel: w56 -> [w74 w79]
        disable-tunnel: [w73 w79] -> w55
        disable-tunnel: [w72 w80] -> w54
        disable-tunnel: [w60 string[] [] ("dmm(s) idn strings")] -> w53
        disable-tunnel: [w59 string[] []] -> w52
        disable-tunnel: w51 -> [w58 _]
        frame condition #0 (active) {
          n11 = Unbundle By Name(w74) -> ("3458A"=w71:T13)
          n12 = call "3458A Initialize Virtual Channels.vi"("error in"=w76, "reset instruments (False)"=w58, "digitizer in"=w71) -> ("error out"=w72:errorcluster, "awg idn string"=w70:string, "dmm(s) idn strings"=w60:string[], "digitizer out"=w75:T13, "sync unit idn string"=w63:string)  [unwired: 4 in]
          n13 = call "3458A Check Needed Aux HW.vi"("digitizer session"=w71) -> ("uses AWG clocking?"=w69:bool, "uses counter?"=w64:bool)  [unwired: 13 in, 4 out]
          n14 = Bundle By Name(cluster=w74, "3458A"=w75) -> (w73:T1)
          n15 = Build Array(w70) -> (w68:string[])
          n16 = Build Array(w63) -> (w65:string[])
          n17 = Select(t=w68, s=w69, f=string[] []) -> (s? t:f=w62:string[])
          n18 = Select(t=w65, s=w64, f=string[] []) -> (s? t:f=w61:string[])
          n19 = Build Array (concatenate)(w62, w61) -> (w59:string[])
        }
        frame condition #1 {
          n20 = xnode "Error Ring"() -> ("error out"=w81:errorcluster)
          n21 = Merge Errors(w82, w81) -> (w80:errorcluster)
        }
      }
    }
    frame "Keysight DSO" {
      n22 = disable-structure shown="w_visa==1" {
        disable-tunnel: w94 -> [w98 w108]
        disable-tunnel: w93 -> [w102 w105]
        disable-tunnel: [w101 w105] -> w92
        disable-tunnel: [w97 w106] -> w91
        disable-tunnel: [w95 string[] [] ("dmm(s) idn strings")] -> w90
        disable-tunnel: [_ string[] []] -> w89
        disable-tunnel: w88 -> [w96 _]
        frame condition #0 (active) {
          n23 = Unbundle By Name(w102) -> ("keysight dso"=w100:T72)
          n24 = call "KeDSO Initialize Virtual Channels.vi"("error in"=w98, "Reset (True)"=w96, "keysight dso"=w100) -> ("error out"=w97:errorcluster, "channel ids"=w95:string[], "keysight dso out"=w99:T72)  [unwired: 6 in]
          n25 = Bundle By Name(cluster=w102, "keysight dso"=w99) -> (w101:T1)
        }
        frame condition #1 {
          n26 = xnode "Error Ring"() -> ("error out"=w107:errorcluster)
          n27 = Merge Errors(w108, w107) -> (w106:errorcluster)
        }
      }
    }
    frame "CMI ADS127L21" {
      n28 = disable-structure shown="w_visa==1" {
        disable-tunnel: w119 -> [w124 w132]
        disable-tunnel: w118 -> [w126 w129]
        disable-tunnel: [w125 w129] -> w117
        disable-tunnel: [w123 w130] -> w116
        disable-tunnel: [w120 string[] [] ("dmm(s) idn strings")] -> w115
        disable-tunnel: [_ string[] []] -> w114
        frame condition #0 (active) {
          n29 = Unbundle By Name(w126) -> ("ADS127L21"=w122:T81)
          n30 = call "CMI ADS127L21 - Config Virtual Channels.vi"("error in (no error)"=w124, "ADS127L21 session"=w122) -> ("error out"=w123:errorcluster, "virtual channel idns"=w120:string[], "ADS127L21 session out"=w121:T81)  [unwired: 6 in, 1 out]
          n31 = Bundle By Name(cluster=w126, "ADS127L21"=w121) -> (w125:T1)
        }
        frame condition #1 {
          n32 = xnode "Error Ring"() -> ("error out"=w131:errorcluster)
          n33 = Merge Errors(w132, w131) -> (w130:errorcluster)
        }
      }
    }
    frame "cDAQ ADC" {
      n34 = disable-structure shown="w_daqmx==1" {
        disable-tunnel: w144 -> [w149 w158]
        disable-tunnel: w143 -> [w152 w155]
        disable-tunnel: [w151 w155] -> w142
        disable-tunnel: [w148 w156] -> w141
        disable-tunnel: [w146 string[] [] ("dmm(s) idn strings")] -> w140
        disable-tunnel: [_ string[] []] -> w139
        disable-tunnel: w138 -> [w147 _]
        frame condition #0 (active) {
          n35 = Unbundle By Name(w152) -> ("cdaq"=w145:T78)
          n36 = call "cDAQ Open ADC.vi"("error in"=w149, "Reset (False)"=w147, "cdaq session in"=w145) -> ("error out"=w148:errorcluster, "channel idns"=w146:string[], "cdaq session out"=w150:T78)  [unwired: 6 in]
          n37 = Bundle By Name(cluster=w152, "cdaq"=w150) -> (w151:T1)
        }
        frame condition #1 {
          n38 = xnode "Error Ring"() -> ("error out"=w157:errorcluster)
          n39 = Merge Errors(w158, w157) -> (w156:errorcluster)
        }
      }
    }
    frame "DirectSound DLL" {
      n40 = Unbundle By Name(w168) -> ("dsdll"=w169:T52)
      n41 = call "DSDLL Initialize Virtual Channels.vi"("error in"=w170, "dsdll session"=w169) -> ("error out"=w166:errorcluster, "channel names"=w164:string[], "dsdll session out"=w167:T52)  [unwired: 6 in, 1 out]
      n42 = Bundle By Name(cluster=w168, "dsdll"=w167) -> (w165:T1)
    }
    frame "dummy", Default {
      n43 = Unbundle By Name(w174) -> ("simadc"=w175:T57)
      n44 = call "SimAdc Initialize Virtual Channels.vi"("error in"=w177, "simadc in"=w175) -> ("error out"=w176:errorcluster, "channel identifiers"=w172:string[], "simadc out"=w173:T57)  [unwired: 7 in]
      n45 = Bundle By Name(cluster=w174, "simadc"=w173) -> (w171:T1)
    }
  }
  n46 = call "MPX Open.vi"("error in"=w3, "session in"=w2) -> ("error out"=→"error out":errorcluster, "idn string"=w8:string, "session out"=w4:T1)  [unwired: 7 in]
  "multiplexer idn string" <- w8
  n47 = Unbundle By Name(w4) -> ("multiplex"=w18:T60)
  n48 = Empty String/Path?(string/path=w8) -> (empty?=w11:bool)
  n49 = Unbundle By Name(w18) -> ("enabled"=w17:bool, "sequence"=w14:string[], "idn string"=w12:string)
  n50 = Build Array (concatenate)(w9, w8) -> (w10:string[])
  n51 = Select(t=w9, s=w11, f=w10) -> (s? t:f=w6:string[])
  "aux instr. idn strings" <- w6
  n52 = Empty Array?(array=w14) -> (empty?=w16:bool)
  n53 = Compound Arithmetic op=AND(w17, invert w16) -> (w15:bool)
  n54 = case shown="True" w15 {
    tunnel: w14 -> [_ w181]
    tunnel: w13 -> [w178 w182]
    tunnel: [w178 w180] -> w7
    tunnel: w12 -> [_ w179]
    frame False {
    }
    frame True {
      n55 = for {
        tunnel: w182 -> [w186]
        tunnel: w181 -> [w185] mode=indexing
        tunnel: [w184] -> w180 mode=concatenating
        tunnel: w179 -> [w183]
        n56 = for {
          tunnel: w186 -> [w190] mode=indexing
          tunnel: w185 -> [w189]
          tunnel: [w188] -> w184 mode=indexing
          tunnel: w183 -> [w187]
          n57 = Format Into String(format string=" | MUX: %s | PATH: %s", initial string=w190, w187, w189) -> (resulting string=w188:string)  [unwired: 1 in, 1 out]
        }
      }
    }
  }
  "channel idn strings" <- w7
  n58 = Bundle By Name(cluster=w4, "channel idn str"=w7, "aux instr idn str"=w6, "accessed?"=TRUE) -> (→"adc session out":T1)
  n59 = Build Array (concatenate)(w7, w6) -> (→"all instruments idn strings":string[])
